vi "Camera.vi"(11 "error in (no error)":errorcluster) -> (1 "Camera 2":bool, 2 "Feature list  3":i32, 3 "Out":bool)   [LabVIEW 2015]
uses:
  Control Button/Exit.ctl
  Control PB/Next_.ctl
panel:
  in  "Feature list":i32(listbox)
  in  "Desontter":bool
  in  "Next":T1
  in  "Exit":T2
  # "Add Feature List"
  # "CAM1"
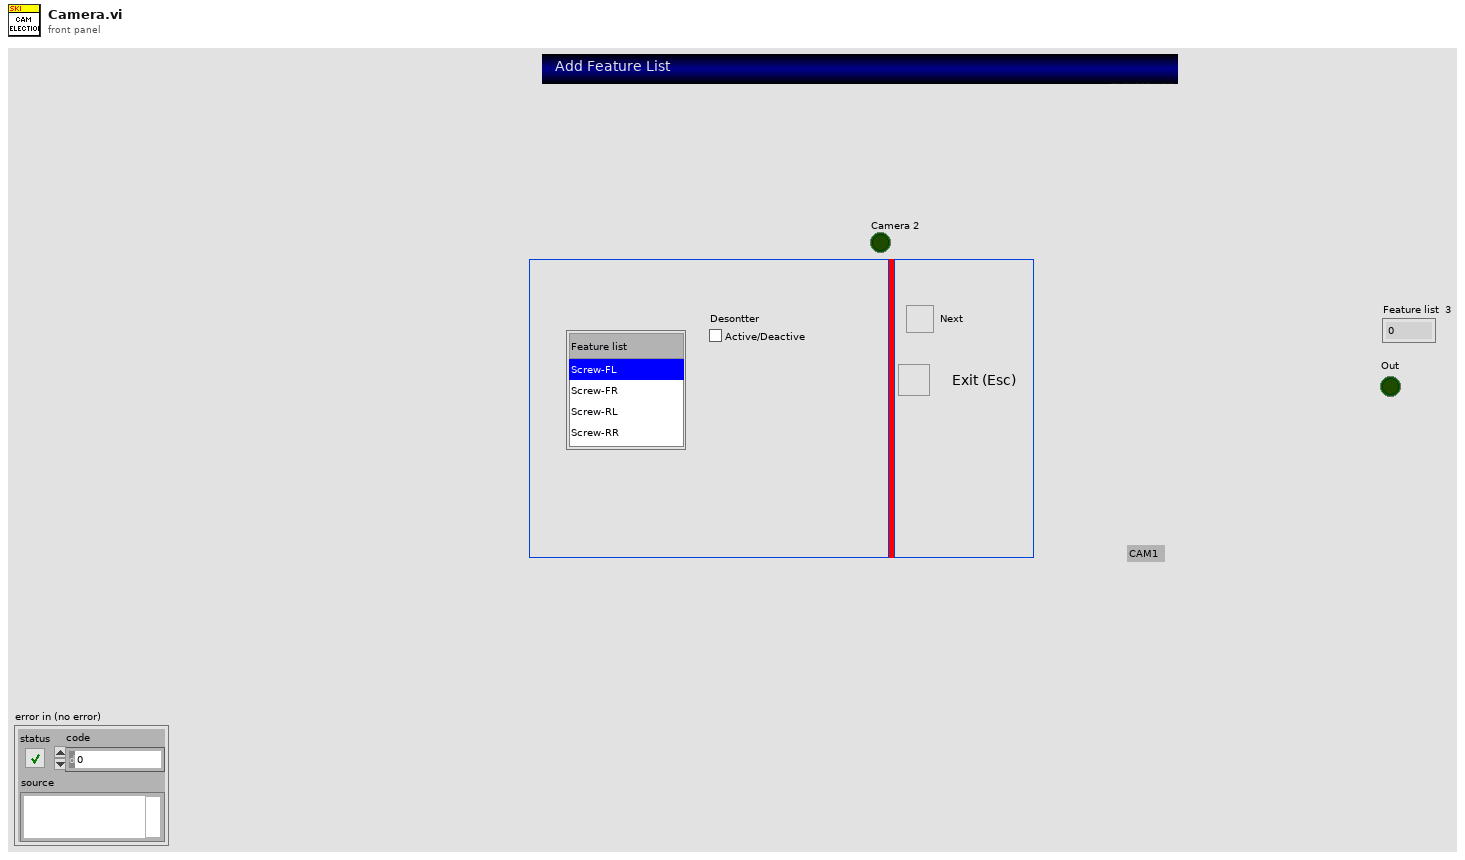
[diagram p1: front panel]
types:
  T1 = typedef "Next_.ctl" = bool
  T2 = typedef "Exit.ctl" = bool
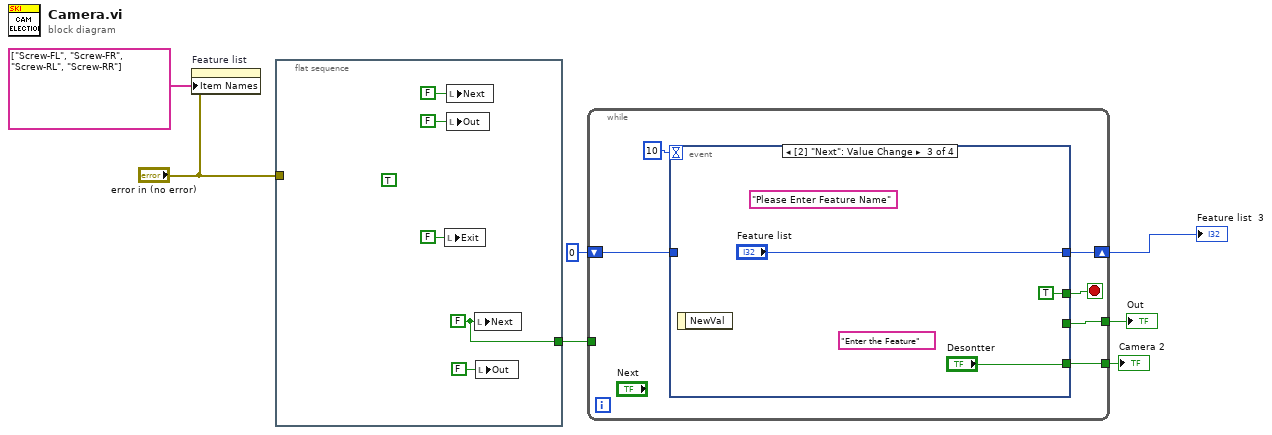
[diagram p0: block diagram]
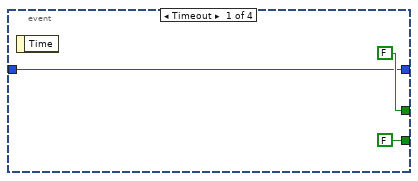
[diagram p2: hidden frame]
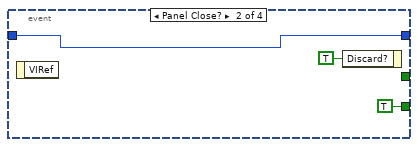
[diagram p3: hidden frame]
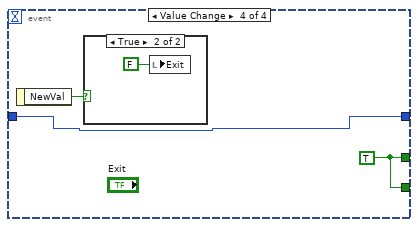
[diagram p4: hidden frame]
diagram:
  n1 = property on="Feature list" class="LstBox (strict)"(error in="error in (no error)", "Item Names"=string[] ["Screw-FL", "Screw-FR", "Screw-RL", "Screw-RR"]) -> ()  [unwired: 1 in, 2 out]
  n2 = flat-sequence {
    tunnel: [w9] -> w6
    tunnel: "error in (no error)" -> [_]
    frame #0 {
      w9 = T1 FALSE ("Next")
      (unwired) TRUE ("Key Focus")
      n3 = local write "Exit"(FALSE ("Exit")) -> ()
      n4 = local write "Next"(T1 FALSE ("Next")) -> ()
      n5 = local write "Out"(FALSE ("Out")) -> ()
      n6 = local write "Next"(w9) -> ()
      n7 = local write "Out"(FALSE ("Out")) -> ()
    }
  }
  n8 = while {
    tunnel: [w17] -> w7
    tunnel: w6 -> [_]
    tunnel: [w15] -> w5
    shift-right: [w14] -> w1
    shift-left: 0 ("Feature list") -> [w13]
    stop <- w18 stop-if-true
    n9 = event shown="[2] \"Next\": Value Change" {
      selector: _ -> [_ _ _ _]
      dyn-events: _ -> [_ _ _ _]
      timeout: 10 -> [_ _ _ _]
      tunnel: [FALSE _ TRUE w29] -> w18
      tunnel: [T1 FALSE ("NewVal") T1 TRUE ("NewVal") _ w29] -> w17
      tunnel: [_ _ "Desontter" _] -> w15
      tunnel: [w19 w22 "Feature list" w28] -> w14
      tunnel: w13 -> [w19 w22 _ w28]
      event Timeout {
        n10 = event-data() -> ()  [unwired: 1 in, 1 out]
      }
      event Panel Close? {
        n11 = event-data() -> ()  [unwired: 1 in, 1 out]
        n12 = event-data("Discard?"=TRUE) -> ()  [unwired: 1 in, 1 out]
      }
      event Value Change {
        (unwired) "Enter the Feature"
        (unwired) "Please Enter Feature Name" ("message")
        n13 = event-data() -> ()  [unwired: 1 in, 1 out]
      }
      event Value Change {
        w29 = TRUE
        n14 = event-data() -> ("NewVal"=w30:T2)  [unwired: 1 in]
        n15 = case shown="True" w30 {
          frame False {
          }
          frame True {
            n16 = local write "Exit"(T1 FALSE ("Next")) -> ()
          }
        }
      }
    }
  }
  "Out" <- w7
  "Camera 2" <- w5
  "Feature list  3" <- w1
